vi "brc_daq_scan_modules.vi"() -> (14 "module_number":i32, 19 "error out":errorcluster)   [LabVIEW 2019, in "BRC-DAQ x86.lvlib"]
uses:
  BRC-DAQ x86.lvlib
  DLL/brc_daq_sdk.dll
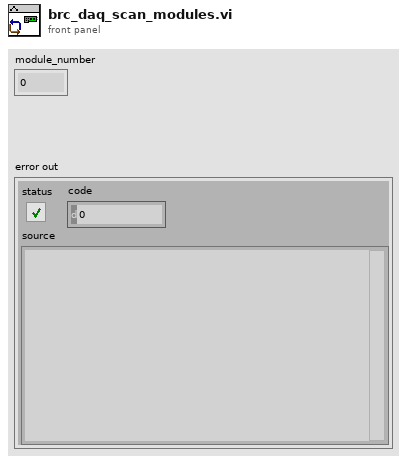
[diagram p1: front panel]
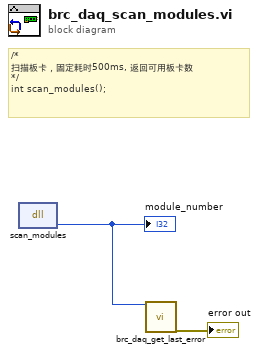
[diagram p0: block diagram]
diagram:
  # "/*\n扫描板卡，固定耗时500ms, 返回可用板卡数\n*/\nint scan_modules();"
  n1 = dll-call lib="E:/01 BRC project/04BRC-daq/04 Drive/BRC-DAQ/DAQ-x64/DLL/brc_daq_sdk.dll" fn="scan_modules"() -> ("return type"=w2:i32)  [unwired: 3 in, 2 out]
  "module_number" <- w2
  n2 = call "brc_daq_get_last_error.vi"("return_value"=w2) -> ("error out"=→"error out":errorcluster)  [unwired: 18 in]
